vi "Counter Setup Delta T Mode.vi"(8 "error in":errorcluster, 11 "counter session in":T1) -> (0 "error out":errorcluster, 3 "counter session out":T1)   [LabVIEW 2013, in "Counter.lvlib"]
doc: "Call this to initialize counter to delta T measurement. Trigger levels are configured for 2V treshold and negative edge."
uses:
  Counter.lvlib
  Counter Session.ctl
  Counter Type.ctl
  Picotest U62XXA/PICOTEST U62XXA series.lvlib
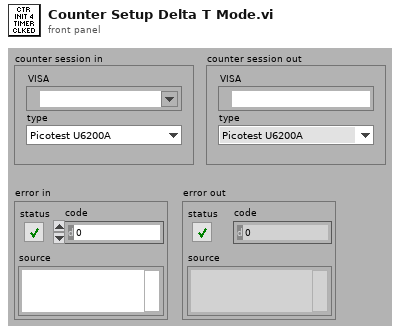
[diagram p1: front panel]
types:
  T1 = typedef "Counter.lvlib/Counter Session.ctl" = cluster{"VISA":refnum<visa-resource-name>, "type":T2}
  T2 = typedef "Counter.lvlib/Counter Type.ctl" = enum16{"Picotest U6200A", "dummy"}
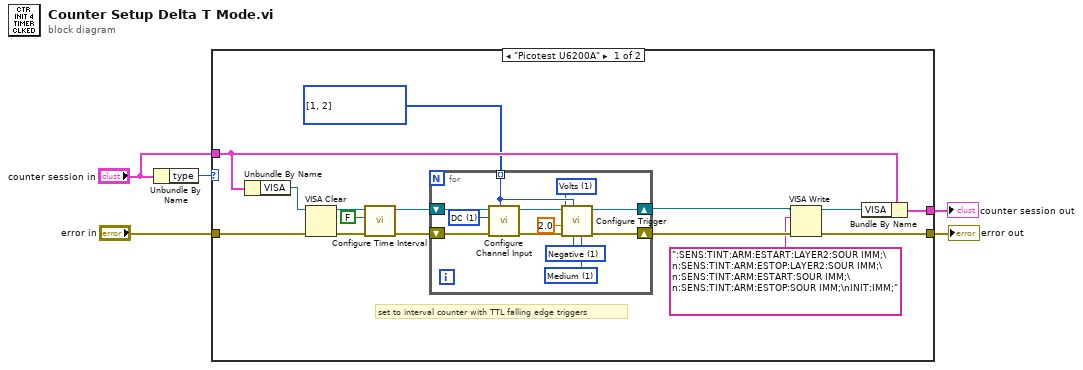
[diagram p0: block diagram]
diagram:
  n1 = Unbundle By Name("counter session in") -> ("type"=w5:T2)
  n2 = case shown="\"Picotest U6200A\"" w5 {
    tunnel: "error in" -> [w15 w34]
    tunnel: "counter session in" -> [w20 w33]
    tunnel: [w17 w34] -> w3
    tunnel: [w19 w33] -> w1
    frame "Picotest U6200A" {
      w18 = i32[] [1, 2] items=["Channel 1"=1, "Channel 2"=2]
      # "set to interval counter with TTL falling edge triggers"
      n3 = Unbundle By Name(w20) -> ("VISA"=w14:refnum<visa-resource-name>)
      n4 = VISA Clear(VISA resource name=w14, error in (no error)=w15) -> (VISA resource name out=w8:refnum<visa-resource-name>, error out=w11:errorcluster)
      n5 = call "Configure Time Interval.vi"("error in (no error)"=w11, "Enable Common (Disable)"=FALSE, "VISA resource name"=w8) -> ("error out"=w10:errorcluster, "VISA resource name out"=w9:refnum<visa-resource-name>)  [unwired: 7 in]
      n6 = for {
        tunnel: w18 -> [w27] mode=indexing
        shift-right: [w22] -> w13
        shift-left: w10 -> [w32]
        shift-right: [w21] -> w12
        shift-left: w9 -> [w31]
        w24 = 1 items=["Percent", "Volts"] ("Trigger Level Type (0:Percent)")
        w25 = 1 items=["High", "Medium", "Low"] ("Sensitivity (0:High)")
        w26 = 1 items=["Positive", "Negative"] ("Trigger Slope (0:Positive)")
        w30 = 1 items=["AC", "DC"] ("Coupling (0:AC)")
        n7 = call "Configure Channel Input.vi"("Channel (1:Channel 1)"=w27, "error in (no error)"=w32, "Coupling (0:AC)"=w30, "VISA resource name"=w31) -> ("error out"=w29:errorcluster, "VISA resource name out"=w28:refnum<visa-resource-name>)  [unwired: 6 in]
        n8 = call "Configure Trigger.vi"("Sensitivity (0:High)"=w25, "Trigger Slope (0:Positive)"=w26, "Channel (1:Channel 1)"=w27, "error in (no error)"=w29, "Trigger Level (50%)"=2.0, "Trigger Level Type (0:Percent)"=w24, "VISA resource name"=w28) -> ("error out"=w22:errorcluster, "VISA resource name out"=w21:refnum<visa-resource-name>)  [unwired: 3 in]
      }
      n9 = VISA Write(VISA resource name=w12, write buffer=":SENS:TINT:ARM:ESTART:LAYER2:SOUR IMM;\n:SENS:TINT:ARM:ESTOP:LAYER2:SOUR IMM;\n:SENS:TINT:ARM:ESTART:SOUR IMM;\n:SENS:TINT:ARM:ESTOP:SOUR IMM;\nINIT:IMM;", error in (no error)=w13) -> (VISA resource name out=w16:refnum<visa-resource-name>, error out=w17:errorcluster)  [unwired: 1 out]
      n10 = Bundle By Name(cluster=w20, "VISA"=w16) -> (w19:T1)
    }
    frame Default {
    }
  }
  "error out" <- w3
  "counter session out" <- w1
